vi "2039_hw OpenTalonDrive.vi"(2 "error in":errorcluster, 3 "refnum name":string="RobotDrive", 4 "CAN IDs":i8[](array[numeric]), 5 "Control Mode":T5) -> (0 "error out":errorcluster, 1 "Drivetrain Talon SRX Ref Array":T1[](array[typedef]))   [LabVIEW 2016]
uses:
  <vilib>/Rock Robotics/WPI/ThirdParty/CanMotor/TalonSRX/WPI_CANTalonSRX_APIControlMode.ctl
  <vilib>/Rock Robotics/WPI/MotorControl/WPI_MotorControlDeviceRef.ctl
  <vilib>/Rock Robotics/WPI/MotorControl/WPI_MotorControlType.ctl
  <vilib>/Rock Robotics/SystemInterfaces/DIO/FPGA_DIOPWMChannel.ctl
  <vilib>/Rock Robotics/WPI/PWM/WPI_PWMDeadband.ctl
  <vilib>/Rock Robotics/WPI/RobotDrive/WPI_RobotDriveOpen4MotorWithExistingMotors.vi
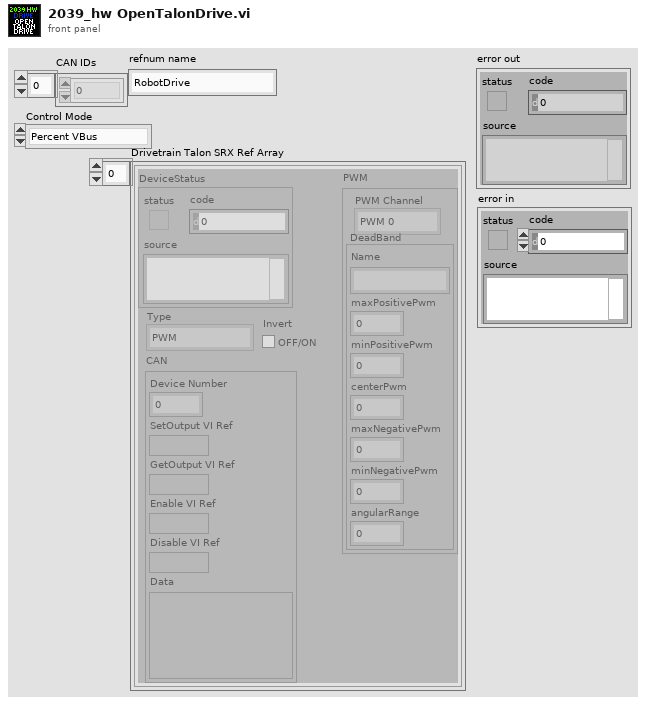
[diagram p1: front panel]
types:
  T1 = typedef "WPI_MotorControlDeviceRef.ctl" = cluster{"DeviceStatus":errorcluster, "Type":T2, "PWM":cluster{"PWM Channel":T3, "DeadBand":T4}, "CAN":cluster{"Device Number":u8, "SetOutput VI Ref":variant, "GetOutput VI Ref":variant, "Enable VI Ref":variant, "Disable VI Ref":variant, "Data":variant}, "Invert":bool}
  T2 = typedef "WPI_MotorControlType.ctl" = enum16{"PWM", "CAN"}
  T3 = typedef "FPGA_DIOPWMChannel.ctl" = enum8{"PWM 0", "PWM 1", "PWM 2", "PWM 3", "PWM 4", "PWM 5", "PWM 6", "PWM 7", "PWM 8", "PWM 9", "PWM MXP 0", "PWM MXP 1", "PWM MXP 2", "PWM MXP 3", "PWM MXP 4", "PWM MXP 5", "PWM MXP 6", "PWM MXP 7", "PWM MXP 8", "PWM MXP 9", "Invalid"}
  T4 = typedef "WPI_PWMDeadband.ctl" = cluster{"Name":string, "maxPositivePwm":i32, "minPositivePwm":i32, "centerPwm":i32, "maxNegativePwm":i32, "minNegativePwm":i32, "angularRange":u16}
  T5 = typedef "WPI_CANTalonSRX_APIControlMode.ctl" = enum8{"Percent VBus", "Speed", "Position", "Slave", "Unchanged / Invalid", "Voltage Compensation", "Current", "Motion Profile", "Motion Magic"}
  T6 = typedef "WPI_RobotDriveDevRef.ctl" = cluster{"DevStatus":errorcluster, "Motors[]":T1[], "Square Inputs":bool, "Max Output":dbl}
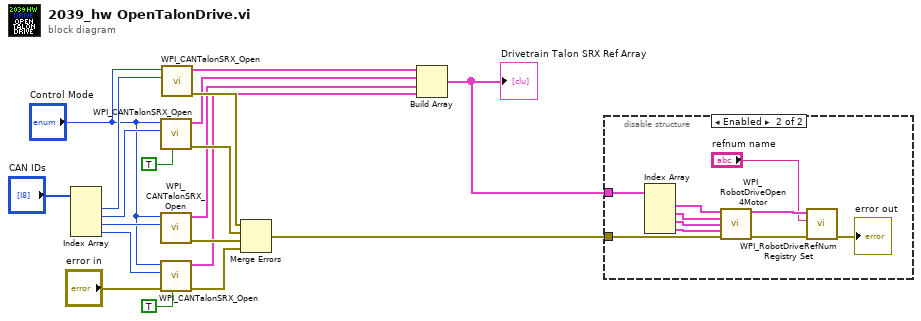
[diagram p0: block diagram]
diagram:
  n1 = Index Array(array="CAN IDs") -> (element #1=w16:i8, element #2=w15:i8, element #3=w14:i8, element #4=w13:i8)  [unwired: 4 in]
  n2 = call <vilib>:"WPI_CANTalonSRX_Open.vi"("Invert"=TRUE, "Device Number"=w15, "Control Mode"="Control Mode") -> ("error out"=w8:errorcluster, "CAN Talon SRX Ref"=w4:T1)  [unwired: 7 in]
  n3 = call <vilib>:"WPI_CANTalonSRX_Open.vi"("Device Number"=w14, "Control Mode"="Control Mode") -> ("error out"=w9:errorcluster, "CAN Talon SRX Ref"=w3:T1)  [unwired: 8 in]
  n4 = call <vilib>:"WPI_CANTalonSRX_Open.vi"("Invert"=TRUE, "error in"="error in", "Device Number"=w13, "Control Mode"="Control Mode") -> ("error out"=w10:errorcluster, "CAN Talon SRX Ref"=w2:T1)  [unwired: 6 in]
  n5 = call <vilib>:"WPI_CANTalonSRX_Open.vi"("Device Number"=w16, "Control Mode"="Control Mode") -> ("error out"=w7:errorcluster, "CAN Talon SRX Ref"=w1:T1)  [unwired: 8 in]
  n6 = Merge Errors(w7, w8, w9, w10) -> (w6:errorcluster)
  n7 = Build Array(w1, w4, w3, w2) -> (w11:T1[])
  "Drivetrain Talon SRX Ref Array" <- w11
  n8 = disable-structure shown="Enabled" {
    disable-tunnel: w11 -> [_ w29]
    disable-tunnel: w6 -> [_ w22]
    frame Disabled {
    }
    frame Enabled {
      n9 = Index Array(array=w29) -> (element #1=w20:T1, element #2=w28:T1, element #3=w27:T1, element #4=w26:T1)  [unwired: 4 in]
      n10 = call-poly <vilib>:"WPI_RobotDriveOpen4Motor.vi"("Rear Left Motor Dev Ref"=w20, "Rear Right Motor Dev Ref"=w28, "Front Left Motor Dev Ref"=w27, "Front Right Motor Dev Ref"=w26, "error in (no error)"=w22) -> ("RobotDriveDevRef"=w24:T6, "error out"=w25:errorcluster)  [unwired: 9 in]
      n11 = call <vilib>:"WPI_RobotDriveRefNum Registry Set.vi"("error in (no error)"=w25, "refnum name"="refnum name", "RobotDriveDevRef"=w24) -> ("error out"=→"error out":errorcluster)  [unwired: 7 in, 1 out]
    }
  }
